vi "First Matched Config File.vi"(6 "pattern(ini by default)":string="*.ini", 8 "Recursively(F)":bool, 11 "Searching Directory":path) -> (3 "Matched Config File":path)   [LabVIEW 2017]
doc: "Searches Searching Directory for the first file matching pattern and returns its path. The default pattern is *.ini, and Recrusively(F) extends the search to subfolders."
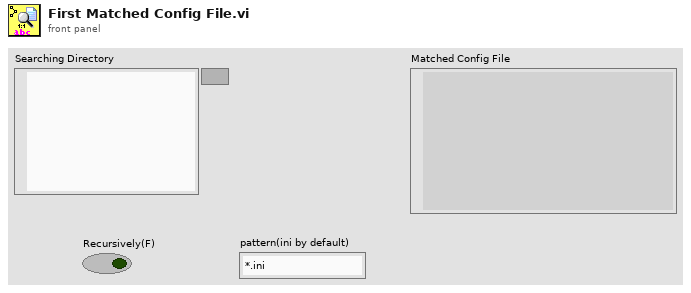
[diagram p1: front panel]
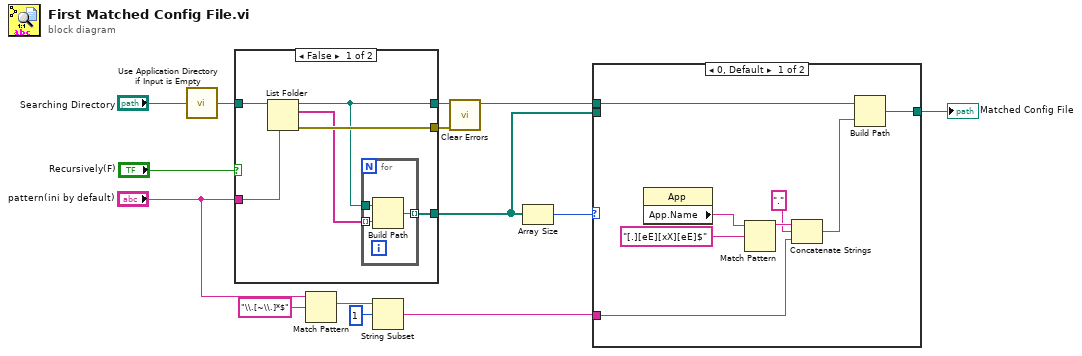
[diagram p0: block diagram]
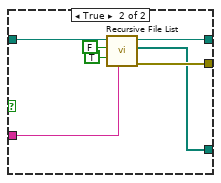
[diagram p2: hidden frame]
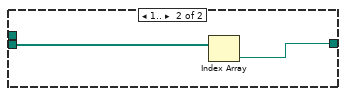
[diagram p3: hidden frame]
diagram:
  n1 = call "Use Application Directory if Input is Empty.vi"("Directory(Use Application Directory if Input is Empty)"="Searching Directory") -> ("Directory"=w11:path)
  n2 = case shown="False" "Recursively(F)" {
    tunnel: [w19 w27] -> w1
    tunnel: "pattern(ini by default)" -> [w17 w25]
    tunnel: w11 -> [w16 w28]
    tunnel: [w15 w26] -> w9
    tunnel: [w14 w29] -> w8
    frame False {
      n3 = List Folder(path=w16, pattern=w17) -> (path out=w14:path, filenames=w18:string[], error out=w19:errorcluster)  [unwired: 2 in, 1 out]
      n4 = for {
        tunnel: w18 -> [w22] mode=indexing
        tunnel: [w21] -> w15 mode=indexing
        tunnel: w14 -> [w20]
        n5 = Build Path(base path=w20, name or relative path=w22) -> (appended path=w21:path)
      }
    }
    frame True {
      n6 = call <vilib>:"Recursive File List.vi"("pattern"=w25, "Continue Recursing on Error? (F)"=TRUE, "Treat LLBs as Folders?"=FALSE, "Folder Path"=w28) -> ("error out"=w27:errorcluster, "All Files in Dir"=w26:path[], "dup Folder Path"=w29:path)  [unwired: 3 in, 2 out]
    }
  }
  n7 = Match Pattern(string="pattern(ini by default)", regular expression="\\.[~\\.]*$") -> (match substring=w6:string)  [unwired: 4 out]
  n8 = String Subset(string=w6, offset (0)=1) -> (substring=w2:string)  [unwired: 1 out]
  n9 = call <vilib>:"Clear Errors.vi"("error in (no error)"=w1) -> ()  [unwired: 5 in, 2 out]
  n10 = Array Size(array=w9) -> (size(s)=w12:i32)
  n11 = case shown="0, Default" w12 {
    tunnel: w9 -> [_ w39]
    tunnel: w8 -> [w37 _]
    tunnel: [w36 w38] -> w13
    tunnel: w2 -> [w30 _]
    frame 0, Default {
      n12 = property class="App"() -> ("App.Name"=w35:string)  [unwired: 2 in, 2 out]
      n13 = Match Pattern(string=w35, regular expression="[.][eE][xX][eE]$") -> (before substring=w33:string)  [unwired: 1 in, 3 out]
      n14 = Concatenate Strings(w33, "." ("string"), w30) -> (w32:string)
      n15 = Build Path(base path=w37, name or relative path=w32) -> (appended path=w36:path)
    }
    frame 1.. {
      n16 = Index Array(array=w39) -> (element=w38:path)  [unwired: 1 in]
    }
  }
  "Matched Config File" <- w13
